vi "qp_map_to_augmented_problem.vi"(8 "error in (no error)":errorcluster, 11 "qp data in":T1) -> (0 "error out":errorcluster, 1 "constrained?":bool, 2 "bounded?":bool, 3 "qp data out":T1)   [LabVIEW 2020, in "NI_Gmath.lvlib"]
uses:
  NI_Gmath.lvlib
  qp_problem data.ctl
  A x Vector.vi
  Create Special Real Matrix.vi
  NI_AALPro.lvlib
  NI_AALBase.lvlib
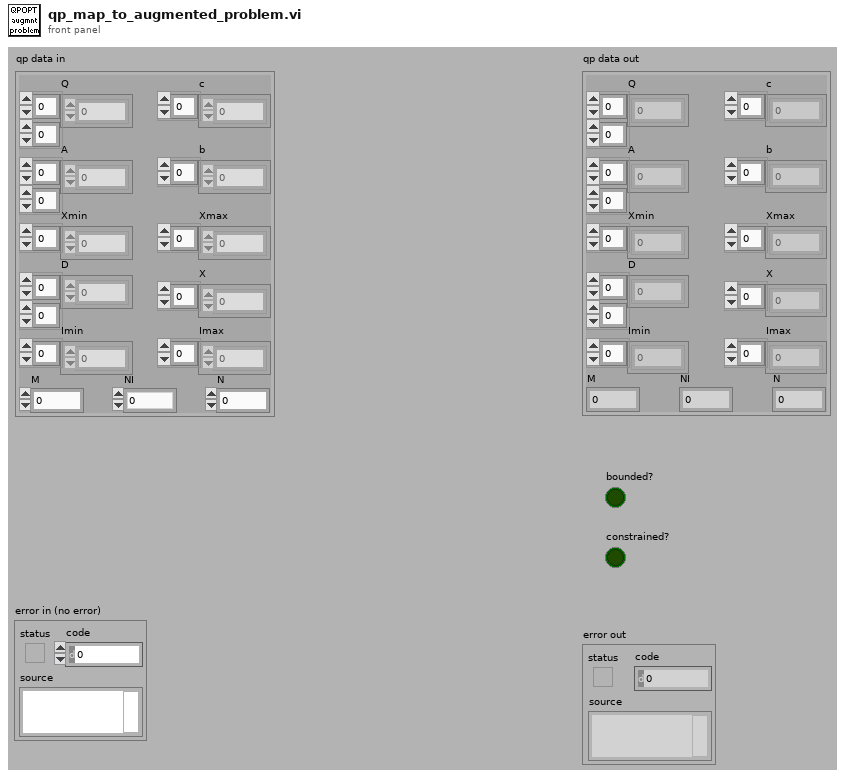
[diagram p1: front panel]
types:
  T1 = typedef "NI_Gmath.lvlib/qp_problem data.ctl" = cluster{"Q":dbl[][], "c":dbl[], "A":dbl[][], "b":dbl[], "Xmin":dbl[], "Xmax":dbl[], "M":i32, "N":i32, "D":dbl[][], "Imax":dbl[], "Imin":dbl[], "NI":i32, "X":dbl[]}
  T2 = typedef "NI_Matrix.lvlib/RealMatrix.ctl" = dbl[][]
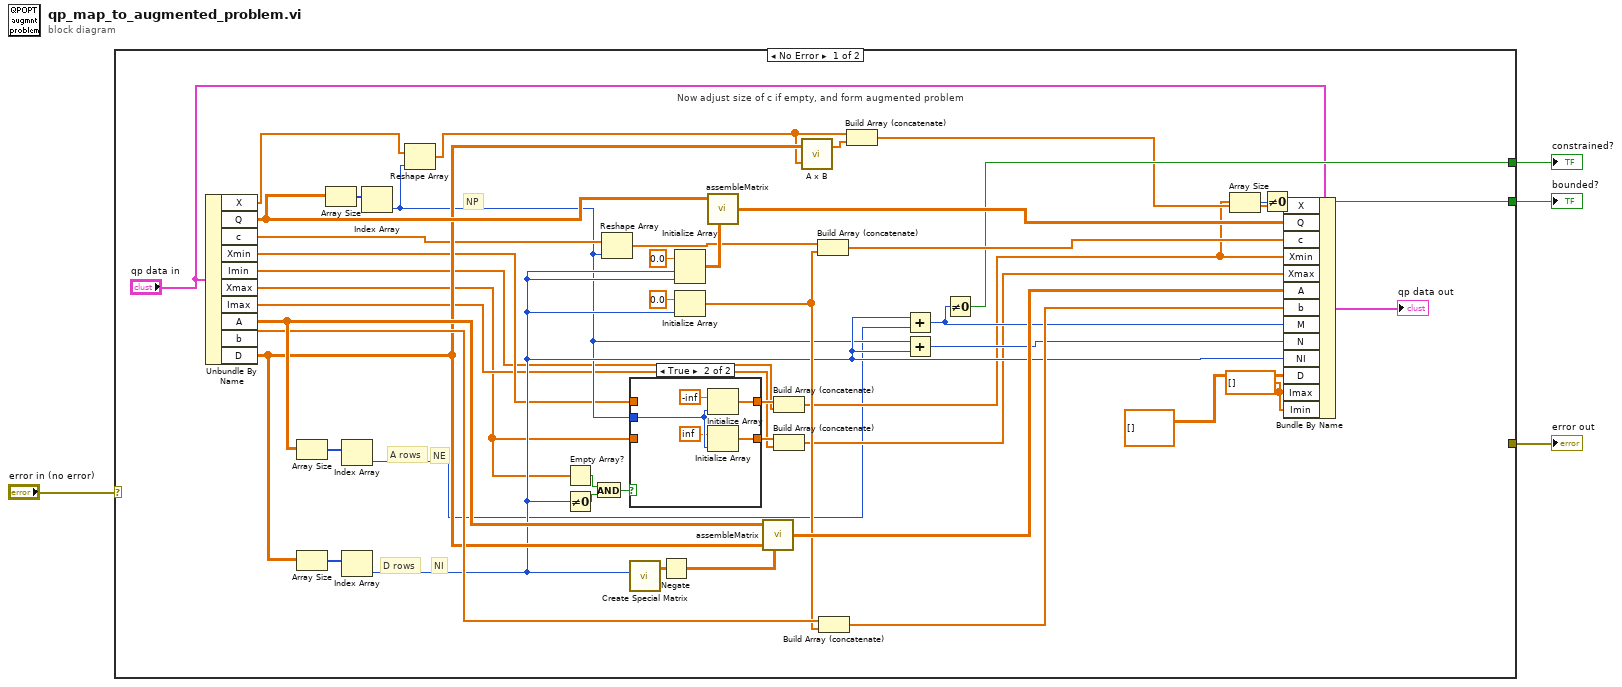
[diagram p0: block diagram]
diagram:
  n1 = case shown="No Error" "error in (no error)" {
    selector: "error in (no error)" -> [_ w58]
    tunnel: [_ w58] -> w1
    tunnel: [w42 _] -> w3
    tunnel: [w43 _] -> w2
    frame No Error {
      w23 = dbl[] [] ("Imax")
      # "Now adjust size of c if empty, and form augmented problem"
      # "NI"
      # "NE"
      # "NP"
      # "D rows"
      # "A rows"
      n2 = Unbundle By Name("qp data in") -> ("X"=w20:dbl[], "Q"=w40:dbl[][], "c"=w26:dbl[], "Xmin"=w11:dbl[], "Imin"=w9:dbl[], "Xmax"=w5:dbl[], "Imax"=w7:dbl[], "A"=w39:dbl[][], "b"=w38:dbl[], "D"=w37:dbl[][])
      n3 = Array Size(array=w39) -> (size(s)=w35:i32[])
      n4 = Array Size(array=w37) -> (size(s)=w36:i32[])
      n5 = Array Size(array=w40) -> (size(s)=w41:i32[])
      n6 = Index Array(array=w35) -> (element=w12:i32)  [unwired: 1 in]
      n7 = Index Array(array=w36) -> (element=w18:i32)  [unwired: 1 in]
      n8 = Index Array(array=w41) -> (element=w15:i32)  [unwired: 1 in]
      n9 = Reshape Array(w20, w15) -> (w21:dbl[])
      n10 = Empty Array?(array=w5) -> (empty?=w6:bool)
      n11 = Not Equal To 0?(x=w18) -> (x != 0?=w17:bool)
      n12 = And(x=w6, y=w17) -> (x .and. y?=w16:bool)
      n13 = Reshape Array(w26, w15) -> (w25:dbl[])
      n14 = case shown="True" w16 {
        tunnel: w15 -> [_ w56]
        tunnel: w11 -> [w52 _]
        tunnel: w5 -> [w51 _]
        tunnel: [w52 w54] -> w10
        tunnel: [w51 w53] -> w8
        frame False {
        }
        frame True {
          n15 = Initialize Array(-inf, w56) -> (w54:dbl[])
          n16 = Initialize Array(inf, w56) -> (w53:dbl[])
        }
      }
      n17 = call-poly "Create Special Matrix.vi"("matrix size"=w18) -> ("Special Matrix"=w24:T2)  [unwired: 4 in, 1 out]
      n18 = Negate(x=w24) -> (-x=w29:T2)
      n19 = Initialize Array(0.0 ("element"), w18, w18) -> (w31:dbl[][])
      n20 = Initialize Array(0.0 ("element"), w18) -> (w33:dbl[])
      n21 = call "assembleMatrix.vi"("A"=w40, "D"=w31) -> ("ABCD"=w50:dbl[][])  [unwired: 3 in]
      n22 = call "assembleMatrix.vi"("A"=w39, "C"=w37, "D"=w29) -> ("ABCD"=w48:dbl[][])  [unwired: 2 in]
      n23 = Build Array (concatenate)(w10, w9) -> (w14:dbl[])
      n24 = Build Array (concatenate)(w8, w7) -> (w13:dbl[])
      n25 = call-poly "A x B.vi"("Vector"=w21, "A"=w37) -> ("A x Vector"=w30:dbl[])  [unwired: 1 out]
      n26 = Build Array (concatenate)(w25, w33) -> (w49:dbl[])
      n27 = Build Array (concatenate)(w38, w33) -> (w47:dbl[])
      n28 = Build Array (concatenate)(w21, w30) -> (w19:dbl[])
      n29 = Add(x=w18, y=w12) -> (x+y=w45:i32)
      n30 = Add(x=w15, y=w18) -> (x+y=w46:i32)
      n31 = Not Equal To 0?(x=w45) -> (x != 0?=w42:bool)
      n32 = Array Size(array=w14) -> (size(s)=w44:i32)
      n33 = Not Equal To 0?(x=w44) -> (x != 0?=w43:bool)
      n34 = Bundle By Name(cluster="qp data in", "X"=w19, "Q"=w50, "c"=w49, "Xmin"=w14, "Xmax"=w13, "A"=w48, "b"=w47, "M"=w45, "N"=w46, "NI"=w18, "D"=dbl[][] [], "Imax"=w23, "Imin"=w23) -> (→"qp data out":T1)
    }
    frame Error {
    }
  }
  "error out" <- w1
  "constrained?" <- w3
  "bounded?" <- w2
